vi "IMAQ-MWT HT TEST without FIFO (HOST).vi"() -> ()   [LabVIEW 2015]
uses:
  <vilib>/FPGAPlugInAG/PCIe-1473R-LX110/niLvFpga_Open_PCIe-1473R-LX110.vi
  <vilib>/rvi/interface/common/dynamic/niFpgaDynamicAddResources.vi
  <vilib>/Utility/error.llb/Error Cluster From Error Code.vi
  <vilib>/rvi/errors/niLvFpgaAdjustHostInterfaceError.vi
  <vilib>/FPGAPlugInAG/Dynamic/niLvFpga_Close_Dynamic.vi
  <vilib>/rvi/interface/nirviOpenFPGA/nirviOpenFPGA.xnode
  FPGA Bitfiles/IMAQ(MWT)_FPGATarget_IMAQ-MWTHTTEST(F_XCRFJH-Ky4E.lvbitx
  <vilib>/rvi/interface/nirviMethod/nirviMethod.xnode
  <vilib>/rvi/interface/nirviReadWriteControl/nirviReadWriteControl.xnode
  <vilib>/rvi/interface/nirviCloseFPGA/nirviCloseFPGA.xnode
  <vilib>/rvi/interface/Simulation/niFpgaSimulationCallBeginRW.vi
  <vilib>/FPGAPlugInAG/Dynamic/niLvFpga_WriteFifo_Dynamic.vi
  <vilib>/rvi/errors/niLvFpgaMergeErrorWithErrorCode.vi
  NiFpgaLv.dll
panel:
  out "Mean Angle":fxp<+/-,32,16> format="%.21g"
  in  "Frame #":i32=40
  out "SPLINE":cluster{u16[], u16[]}(graph)
  out "Frame #":i32
  in  "Loop Interval":u32=1000
  in  "Stop Button":bool
  out "N Points":u16
  out "V2 (ID)":i32
  out "V1 (ID)":i32
  out "Contour":cluster{u16[], u16[]}(graph)
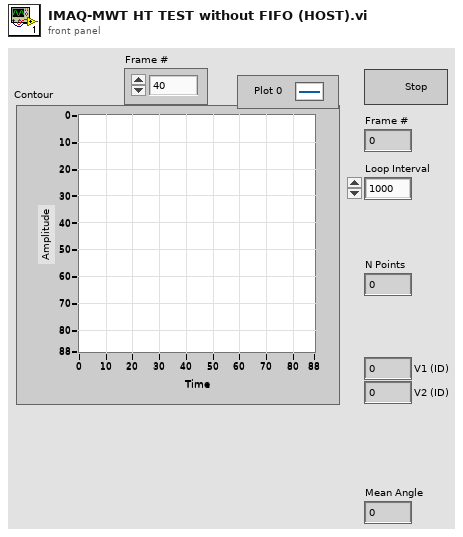
[diagram p1: front panel]
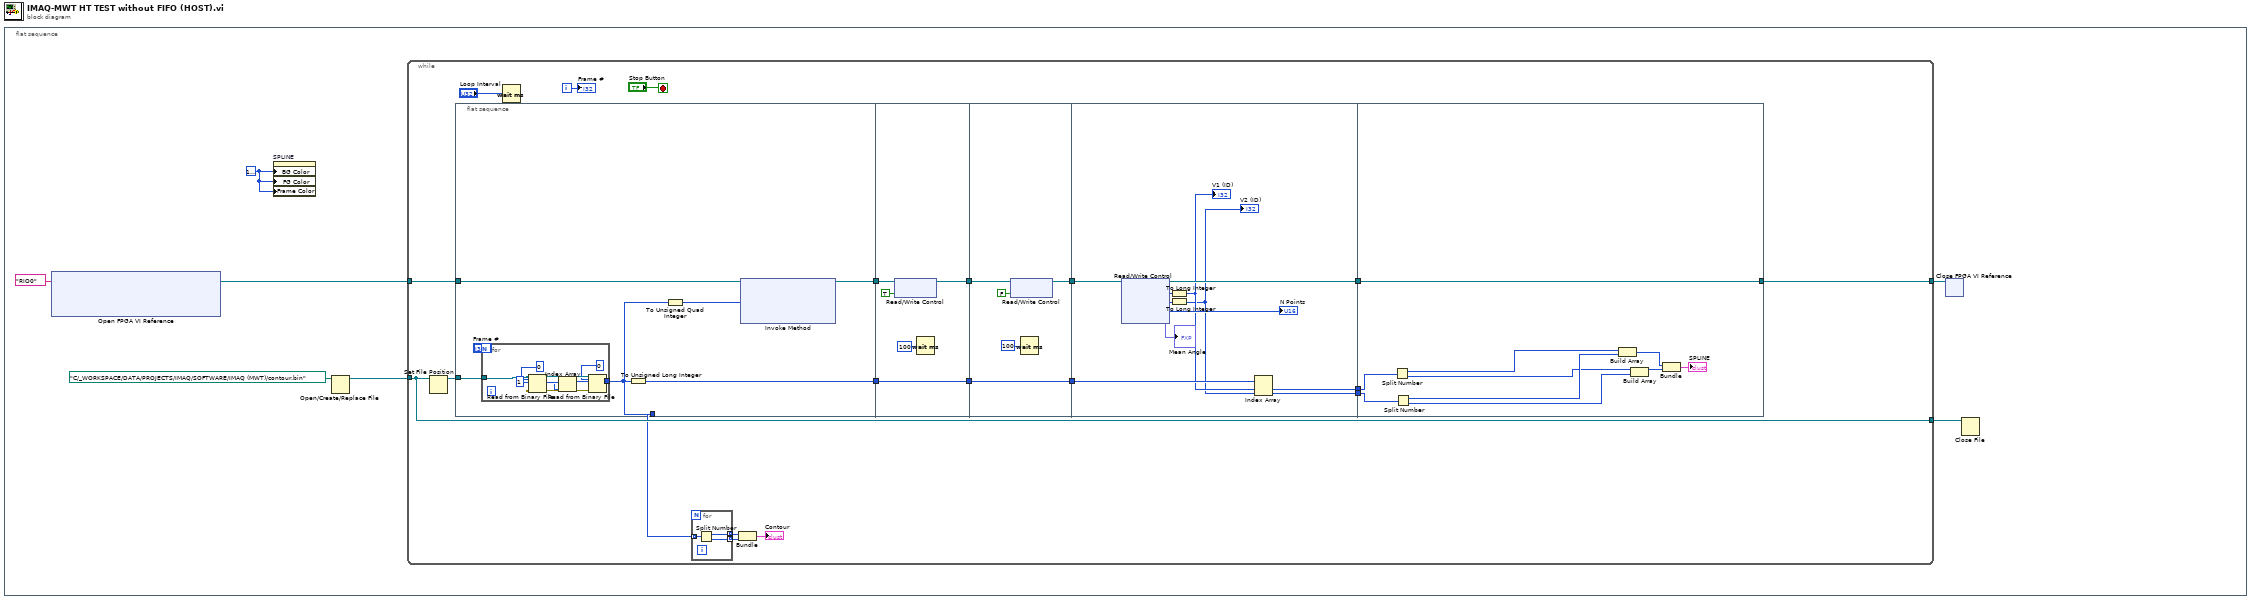
[diagram p0: block diagram]
diagram:
  n1 = flat-sequence {
    frame #0 {
      w2 = u32 16777216 ("Plot Area:Colors:BG Color")
      n2 = xnode "Open FPGA VI Reference"("resource name"=tag "RIO0") -> ("FPGA VI Reference Out"=w1:refnum<k20>)  [unwired: 1 in, 1 out]
      n3 = property on="SPLINE" class="XYGraph (strict)"("BG Color"=w2, "FG Color"=w2, "Frame Color"=w2) -> ()  [unwired: 2 in, 2 out]
      n4 = Open/Create/Replace File(file path (use dialog)=path "C:/_WORKSPACE/DATA/PROJECTS/IMAQ/SOFTWARE/IMAQ (MWT)/contour.bin") -> (refnum out=w5:refnum<file>)  [unwired: 5 in, 2 out]
      n5 = while {
        tunnel: w1 -> [w27]
        tunnel: [w23] -> w6
        tunnel: w5 -> [w21]
        tunnel: [w21] -> w4
        i -> [w14]
        stop <- "Stop Button" stop-if-true
        n6 = Set File Position(refnum=w21) -> (refnum out=w8:refnum<file>)  [unwired: 3 in, 1 out]
        n7 = flat-sequence {
          tunnel: w27 -> [w37]
          tunnel: [w36] -> w26
          tunnel: w8 -> [w35]
          tunnel: [w32] -> w16
          tunnel: [w32] -> w11
          tunnel: w26 -> [w51]
          tunnel: [w49] -> w25
          tunnel: [w47] -> w12
          tunnel: w11 -> [w47]
          tunnel: w25 -> [w56]
          tunnel: [w55] -> w24
          tunnel: [w52] -> w13
          tunnel: w12 -> [w52]
          tunnel: w24 -> [w67]
          tunnel: [w66] -> w15
          tunnel: w13 -> [w64]
          tunnel: [w61] -> w10
          tunnel: [w60] -> w9
          tunnel: [w68] -> w23
          tunnel: w15 -> [w68]
          tunnel: w10 -> [w73]
          tunnel: w9 -> [w72]
          frame #0 {
            n8 = for {
              N: "Frame #" -> [_]
              tunnel: w35 -> [w46]
              tunnel: [w38] -> w33
              n9 = Read from Binary File(5:0 ("count (1)"), 10:1 ("count (1)"), 11:w46) -> (0:w44:errorcluster, 2:w41:i32[], 3:w43:refnum<file>)  [unwired: 3 in, 1 out]
              n10 = Index Array(array=w41) -> (element=w40:i32)  [unwired: 1 in]
              n11 = Read from Binary File(5:u64 0 ("count (1)"), 8:w44, 10:w40, 11:w43) -> (2:w38:u64[])  [unwired: 2 in, 3 out]
            }
            n12 = To Unsigned Long Integer(number=w33) -> (unsigned 32bit integer=w32:u32[])
            n13 = To Unsigned Quad Integer(1:w32) -> (0:w31:u64[])
            n14 = xnode "Invoke Method"("FPGA VI Reference In"=w37, "Data"=w31) -> ("FPGA VI Reference Out"=w36:refnum<k20>)  [unwired: 2 in, 2 out]
          }
          frame #1 {
            n15 = xnode "Read/Write Control"("FPGA VI Reference In"=w51, "Scan End?"=TRUE) -> ("FPGA VI Reference Out"=w49:refnum<k20>)  [unwired: 1 in, 1 out]
            n16 = Wait (ms)(milliseconds to wait=u32 100) -> ()  [unwired: 1 out]
          }
          frame #2 {
            n17 = xnode "Read/Write Control"("FPGA VI Reference In"=w56, "Scan End?"=FALSE) -> ("FPGA VI Reference Out"=w55:refnum<k20>)  [unwired: 1 in, 1 out]
            n18 = Wait (ms)(milliseconds to wait=u32 100) -> ()  [unwired: 1 out]
          }
          frame #3 {
            n19 = xnode "Read/Write Control"("FPGA VI Reference In"=w67) -> ("FPGA VI Reference Out"=w66:refnum<k20>, "V1 (ID)"=w63:u16, "V2 (ID)"=w62:u16, "N Points"=→"N Points":u16, "Mean Angle"=→"Mean Angle":fxp<+/-,32,16>)  [unwired: 1 in, 1 out]
            n20 = To Long Integer(number=w63) -> (32bit integer=w59:i32)
            "V1 (ID)" <- w59
            n21 = To Long Integer(number=w62) -> (32bit integer=w58:i32)
            "V2 (ID)" <- w58
            n22 = Index Array(array=w64, index #1=w59, index #2=w58) -> (element #1=w61:u32, element #2=w60:u32)
          }
          frame #4 {
            n23 = Split Number(x=w73) -> (hi(x)=w77:u16, lo(x)=w75:u16)
            n24 = Split Number(x=w72) -> (hi(x)=w76:u16, lo(x)=w74:u16)
            n25 = Build Array(w77, w76) -> (w70:u16[])
            n26 = Build Array(w75, w74) -> (w69:u16[])
            n27 = Bundle(w70, w69) -> (→"SPLINE":cluster{u16[], u16[]})  [unwired: 1 in]
          }
        }
        n28 = Wait (ms)(milliseconds to wait="Loop Interval") -> ()  [unwired: 1 out]
        n29 = for {
          tunnel: w16 -> [w30] mode=indexing
          tunnel: [w29] -> w18 mode=indexing
          tunnel: [w28] -> w19 mode=indexing
          n30 = Split Number(x=w30) -> (hi(x)=w29:u16, lo(x)=w28:u16)
        }
        n31 = Bundle(w18, w19) -> (→"Contour":cluster{u16[], u16[]})  [unwired: 1 in]
        "Frame #" <- w14
      }
      n32 = xnode "Close FPGA VI Reference"("FPGA VI Reference In"=w6) -> ()  [unwired: 1 in, 1 out]
      n33 = Close File(refnum=w4) -> ()  [unwired: 1 in, 2 out]
    }
  }
